vi "Averager.vi"(1 "b":dbl, 2 "a":dbl) -> (0 "(a+b)/2":dbl)   [LabVIEW 2020]
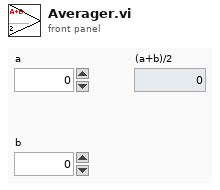
[diagram p1: front panel]
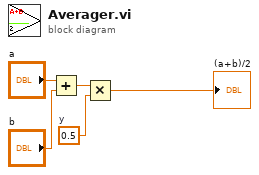
[diagram p0: block diagram]
diagram:
  w4 = 0.5  # y
  n1 = Add(x="a", y="b") -> (x+y=w3:dbl)
  n2 = Multiply(x=w3, y=w4) -> (x*y=→"(a+b)/2":dbl)
